vi "unload File.vi"(8 "error in (no error)":errorcluster, 10 "Path":path, 11 "CSM-Static-Variable-Manager in":refnum<class "CSM-Static-Variable-Manager.lvclass">) -> (0 "error out":errorcluster, 3 "CSM-Static-Variable-Manager out":refnum<class "CSM-Static-Variable-Manager.lvclass">)   [LabVIEW 2017, in "INI-Static-Variable-Support.lvlib" / "CSM-Static-Variable-Manager.lvclass"]
uses:
  CSM-Static-Variable-Manager.lvclass
  CSM-Static-Variable-Manager.lvclass/CSM-Static-Variable-Manager.ctl
  LabVIEW-Config/LabVIEW-Config.lvclass
  <userlib>/_NEVSTOP/Communicable State Machine(CSM)/Communicable State Machine.lvlib
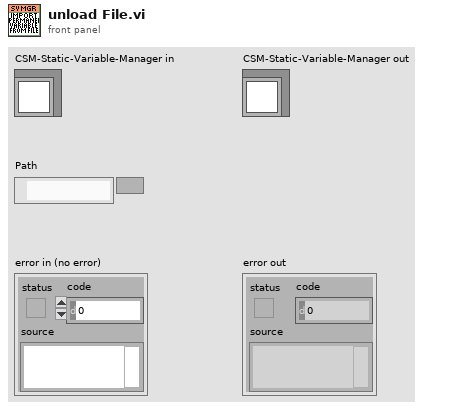
[diagram p1: front panel]
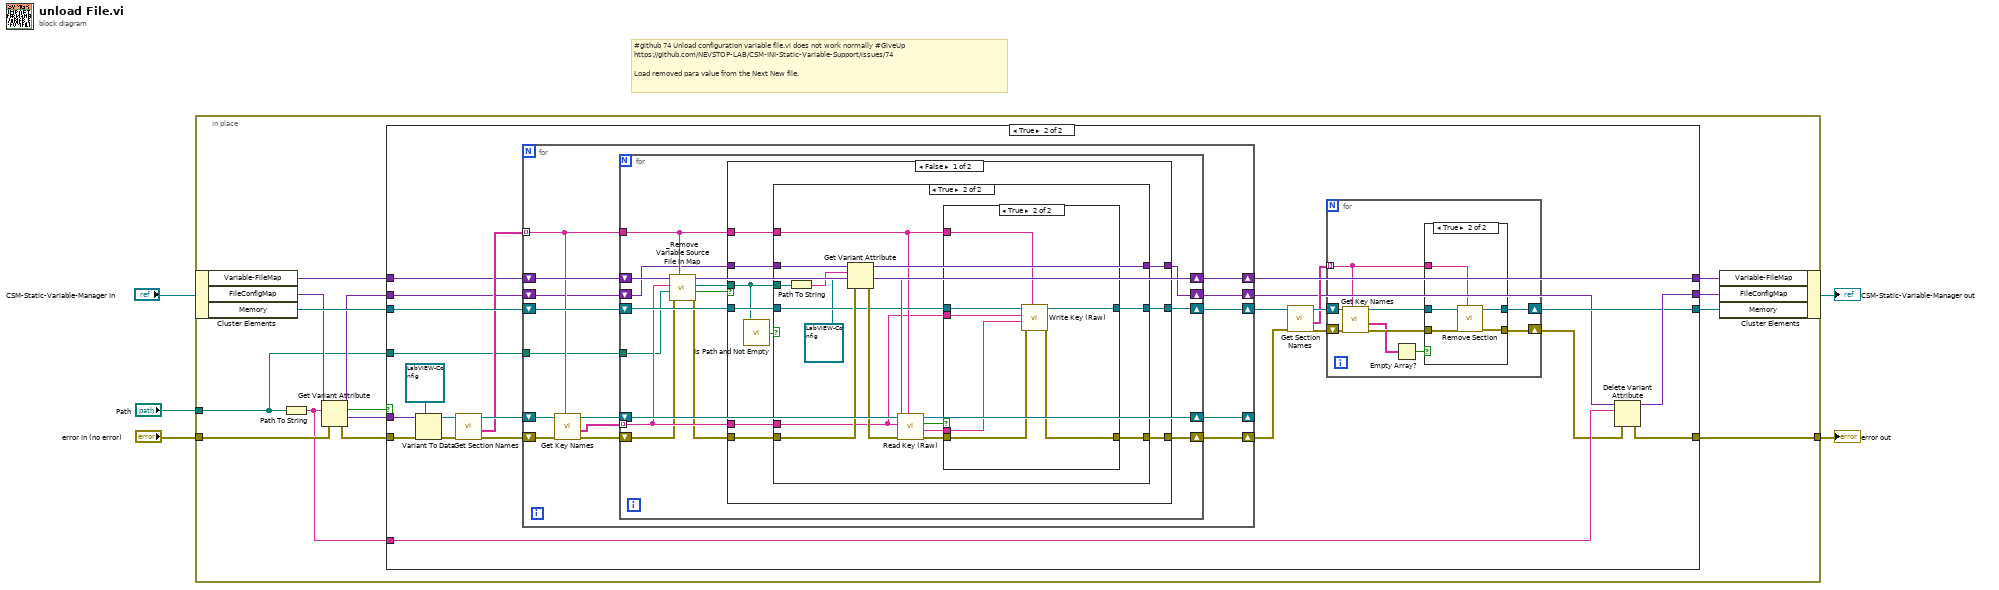
[diagram p0: block diagram]
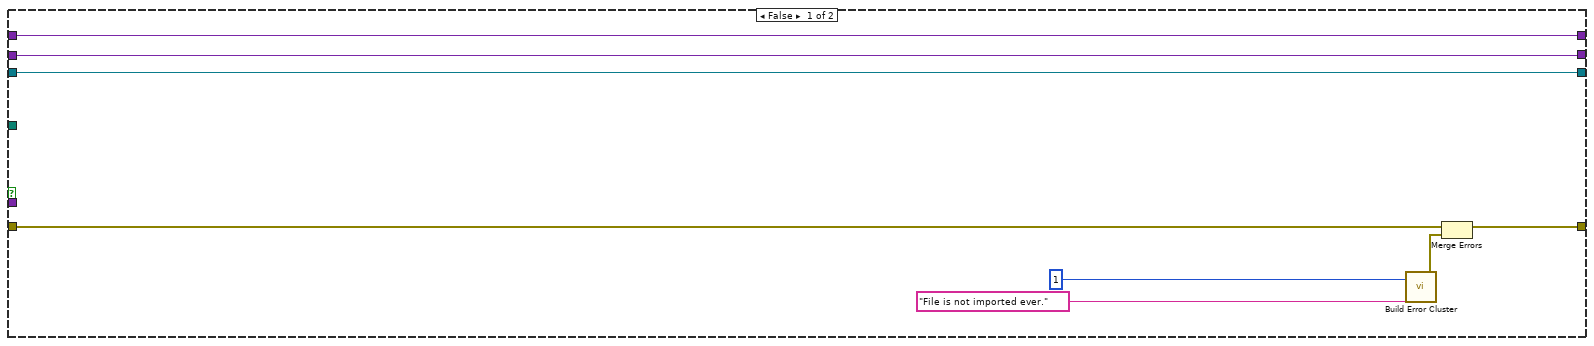
[diagram p2: hidden frame]
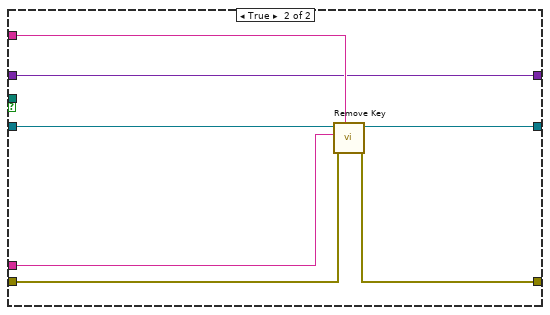
[diagram p6: hidden frame]
diagram:
  # "#github 74 Unload configuration variable file.vi does not work normally #GiveUp\nhttps://github.com/NEVSTOP-LAB/CSM-INI-Static-Variable-Support/issues/74\n\nLoad removed para value from the Next New file."
  n1 = in-place {
    in-place-border: "error in (no error)" -> [w14]
    in-place-border: [w13] -> w2
    in-place-border: "Path" -> [w6]
    n2 = in-place-cluster #1("CSM-Static-Variable-Manager in") -> ("Variable-FileMap"=w9:variant, "FileConfigMap"=w17:variant, "Memory"=w19:refnum<class "LabVIEW-Config.lvclass">)
    n3 = Path To String(path=w6) -> (string=w7:string)
    n4 = Get Variant Attribute(Variant=w17, name=w7, error in=w14) -> (duplicate Variant=w12:variant, found=w10:bool, value=w16:variant, error out=w15:errorcluster)  [unwired: 1 in]
    n5 = case shown="True" w10 {
      tunnel: w19 -> [w26 w51]
      tunnel: [w26 w34] -> w18
      tunnel: w16 -> [_ w50]
      tunnel: w15 -> [w25 w49]
      tunnel: [w24 w46] -> w13
      tunnel: w12 -> [w27 w30]
      tunnel: [w27 w45] -> w11
      tunnel: w9 -> [w20 w40]
      tunnel: [w20 w39] -> w8
      tunnel: w7 -> [_ w41]
      tunnel: w6 -> [_ w38]
      frame False {
        n6 = call <userlib>:"Build Error Cluster.vi"("String to Prepend to source (\"\")"="File is not imported ever." ("String to Prepend to source (\"\")"), "code"=1) -> ("error out"=w23:errorcluster)
        n7 = Merge Errors(w25, w23) -> (w24:errorcluster)
      }
      frame True {
        n8 = Variant To Data(error in=w49, type=refnum<class "LabVIEW-Config.lvclass"> refnum ("LabVIEW-Config.lvlib:LabVIEW-Config.lvclass"), Variant=w50) -> (data=w47:refnum<class "LabVIEW-Config.lvclass">, error out=w48:errorcluster)
        n9 = call "Get Section Names.vi"("error in (no error)"=w48, "Config in"=w47) -> ("error out"=w43:errorcluster, "Section Names"=w42:string[], "Config out"=w44:refnum<class "LabVIEW-Config.lvclass">)  [unwired: 7 in]
        n10 = for {
          shift-right: [w79] -> w35
          shift-left: w51 -> [w80]
          shift-right: [w78] -> w33
          shift-left: w43 -> [w76]
          tunnel: w42 -> [w72] mode=indexing
          shift-right: [w75] -> _
          shift-left: w44 -> [w77]
          shift-right: [w74] -> w39
          shift-left: w40 -> [w73]
          tunnel: w38 -> [w70]
          shift-right: [w68] -> w29
          shift-left: w30 -> [w69]
          n11 = call "Get Key Names.vi"("Section Name"=w72, "error in (no error)"=w76, "Config in"=w77) -> ("error out"=w71:errorcluster, "Key Names"=w81:string[], "Config out"=w82:refnum<class "LabVIEW-Config.lvclass">)  [unwired: 5 in, 1 out]
          n12 = for {
            tunnel: w72 -> [w91]
            tunnel: w81 -> [w90] mode=indexing
            shift-right: [w94] -> w78
            shift-left: w71 -> [w89]
            shift-right: [w97] -> w79
            shift-left: w80 -> [w96]
            shift-right: [w95] -> w75
            shift-left: w82 -> [w95]
            shift-right: [w92] -> w74
            shift-left: w73 -> [w93]
            tunnel: w70 -> [w87]
            shift-right: [w84] -> w68
            shift-left: w69 -> [w85]
            n13 = call "_Remove Variable Source File in Map.vi"("String"=w91, "error in (no error)"=w89, "dup path"=w87, "Content"=w90, "Variable-FileMap"=w93) -> ("error out"=w88:errorcluster, "No Source Any More?"=w86:bool, "Latest File Path (If changed)"=w83:path, "Variant"=w92:variant)  [unwired: 3 in]
            n14 = case shown="False" w86 {
              tunnel: [w103 w142] -> w97
              tunnel: w96 -> [w104 w141]
              tunnel: [w100 w140] -> w94
              tunnel: w91 -> [w102 w139]
              tunnel: w90 -> [w101 w138]
              tunnel: w88 -> [w106 w137]
              tunnel: w85 -> [w107 w136]
              tunnel: [w105 w136] -> w84
              tunnel: w83 -> [w99 _]
              frame False {
                n15 = call <vilib>:"Is Path and Not Empty.vi"("path"=w99) -> ("Is Path and Not Empty?"=w98:bool)  [unwired: 4 in]
                n16 = case shown="True" w98 {
                  tunnel: w107 -> [w110 w126]
                  tunnel: w106 -> [w108 w125]
                  tunnel: [w110 w124] -> w105
                  tunnel: w104 -> [w109 w121]
                  tunnel: [w109 w120] -> w103
                  tunnel: w102 -> [_ w119]
                  tunnel: w101 -> [_ w116]
                  tunnel: [w108 w114] -> w100
                  tunnel: w99 -> [_ w112]
                  frame False {
                  }
                  frame True {
                    n17 = Path To String(path=w112) -> (string=w113:string)
                    n18 = Get Variant Attribute(Variant=w126, name=w113, default value (empty Variant)=refnum<class "LabVIEW-Config.lvclass"> refnum ("LabVIEW-Config.lvlib:LabVIEW-Config.lvclass"), error in=w125) -> (duplicate Variant=w124:variant, value=w123:refnum<class "LabVIEW-Config.lvclass">, error out=w122:errorcluster)  [unwired: 1 out]
                    n19 = call "Read Key (Raw).vi"("Section Name"=w119, "error in (no error)"=w122, "Key Name"=w116, "Config in"=w123) -> ("error out"=w115:errorcluster, "Content"=w117:string, "Key Found?"=w118:bool)  [unwired: 4 in, 1 out]
                    n20 = case shown="True" w118 {
                      tunnel: w121 -> [w128 w135]
                      tunnel: [w128 w134] -> w120
                      tunnel: w119 -> [_ w133]
                      tunnel: w117 -> [_ w131]
                      tunnel: w116 -> [_ w132]
                      tunnel: w115 -> [w127 w130]
                      tunnel: [w127 w129] -> w114
                      frame False {
                      }
                      frame True {
                        n21 = call "Write Key (Raw).vi"("Section Name"=w133, "error in (no error)"=w130, "Content"=w131, "Key Name"=w132, "Config in"=w135) -> ("error out"=w129:errorcluster, "Config out"=w134:refnum<class "LabVIEW-Config.lvclass">)  [unwired: 4 in, 1 out]
                      }
                    }
                  }
                }
              }
              frame True {
                n22 = call "Remove Key.vi"("Section Name"=w139, "error in (no error)"=w137, "Key Name"=w138, "Config in"=w141) -> ("error out"=w140:errorcluster, "Config out"=w142:refnum<class "LabVIEW-Config.lvclass">)  [unwired: 5 in, 1 out]
              }
            }
          }
        }
        n23 = call "Get Section Names.vi"("error in (no error)"=w33, "Config in"=w35) -> ("error out"=w36:errorcluster, "Section Names"=w31:string[], "Config out"=w37:refnum<class "LabVIEW-Config.lvclass">)  [unwired: 7 in]
        n24 = for {
          shift-right: [w54] -> w34
          shift-left: w37 -> [w60]
          shift-right: [w53] -> w32
          shift-left: w36 -> [w57]
          tunnel: w31 -> [w52] mode=indexing
          n25 = call "Get Key Names.vi"("Section Name"=w52, "error in (no error)"=w57, "Config in"=w60) -> ("error out"=w58:errorcluster, "Key Names"=w56:string[], "Config out"=w59:refnum<class "LabVIEW-Config.lvclass">)  [unwired: 5 in, 1 out]
          n26 = Empty Array?(array=w56) -> (empty?=w55:bool)
          n27 = case shown="True" w55 {
            tunnel: w59 -> [w62 w67]
            tunnel: w58 -> [w61 w66]
            tunnel: [w62 w65] -> w54
            tunnel: [w61 w64] -> w53
            tunnel: w52 -> [_ w63]
            frame False {
            }
            frame True {
              n28 = call "Remove Section.vi"("Section Name"=w63, "error in (no error)"=w66, "Config in"=w67) -> ("error out"=w64:errorcluster, "Config out"=w65:refnum<class "LabVIEW-Config.lvclass">)  [unwired: 6 in, 1 out]
            }
          }
        }
        n29 = Delete Variant Attribute(4:w32, 6:w41, 7:w29) -> (0:w46:errorcluster, 3:w45:variant)  [unwired: 1 out]
      }
    }
    n30 = in-place-cluster #1("Variable-FileMap"=w8, "FileConfigMap"=w11, "Memory"=w18) -> (→"CSM-Static-Variable-Manager out":refnum<class "CSM-Static-Variable-Manager.lvclass">)
  }
  "error out" <- w2
